vi "延时.vi"(8 "错误in":errorcluster caption="错误常量", 11 "等待时间（毫秒）":u32) -> (0 "错误in":errorcluster caption="错误常量")   [LabVIEW 2014]
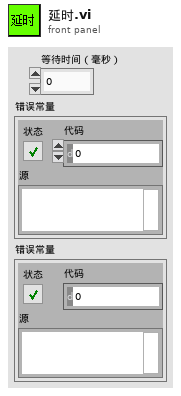
[diagram p1: front panel]
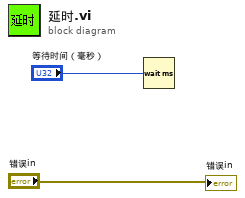
[diagram p0: block diagram]
diagram:
  n1 = Wait (ms)(milliseconds to wait="等待时间（毫秒）") -> ()  [unwired: 1 out]
  "错误in" <- "错误in"
